vi "Process data first.vi"() -> ()   [LabVIEW 2021]
uses:
  <vilib>/Platform/TimedLoop/XDataNode/timing_clust.ctl
  <vilib>/Platform/TimedLoop/XDataNode/nitl_modes.ctl
  <vilib>/Platform/TimedLoop/XDataNode/wakeup.ctl
  <vilib>/picture/3D Picture Control/Object/Create Object (drawable).vi
  <vilib>/picture/3D Picture Control/Object/Add Object (no reference).vi
  <vilib>/picture/3D Picture Control/Object/Add Object (reference).vi
  <vilib>/platform/TimedLoop/XDataNode/XDataNode.xnode
  <vilib>/Platform/TimedLoop/XDataNode/XDNodeRunTimeDep.lvlib
  <vilib>/picture/3D Picture Control/NI_3D Picture Control.lvlib
panel:
  in  "Relative?":bool
  out "output variable 4":dbl
  out "Angle":dbl
  out "output variable 3":dbl
  out "output variable 2":dbl
  out "output variable":dbl
  out "3D Picture":refnum<vi>(3d-picture)
  out "ZRoll":dbl
  out "YRoll":dbl
  out "XRoll":dbl
  in  "stop":bool
  in  "DAQ Port":refnum<visa-resource-name>
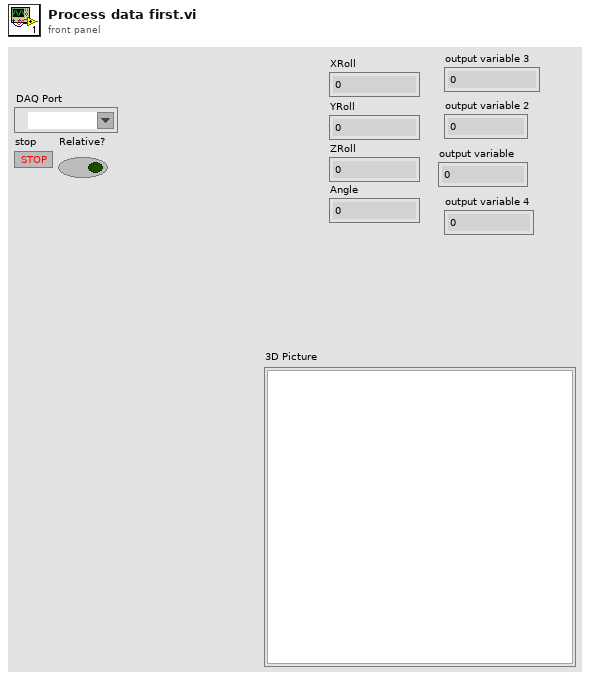
[diagram p1: front panel]
types:
  T1 = cluster{"Red":sgl, "Green":sgl, "Blue":sgl, "Alpha":sgl}
  T2 = typedef "XDNodeRunTimeDep.lvlib/timing_clust.ctl" = cluster{"Expected End [f-1]":u64, "Actual End [f-1]":u64, "Finished Late? [f-1]":bool, "Expected End [i-1]":u64, "Actual End [i-1]":u64, "Finished Late? [i-1]":bool, "Expected Start [i]":u64, "Actual Start [i]":u64, "Expected Start [f]":u64, "Actual Start [f]":u64, "Source Name":string, "Structure Name":string, "Period":i64, "Deadline":i64, "Offset":i64, "Start":i64, "Priority":i32, "Timeout":i32, "Mode":T3, "Wakeup Reason":T4, "Error":errorcluster, "Source Type":string, "Secondary Source Type":string, "Global End Time":u64, "Global Start Time":u64, "Frame Duration":u64, "Iteration Duration":u64, "Assigned CPU":i32, "I/O Scan Engine Mode":u32}
  T3 = typedef "XDNodeRunTimeDep.lvlib/nitl_modes.ctl" = enum32{"No Change", "Process missed periods, maintain original phase", "Discard missed periods, maintain original phase", "Process missed periods, ignore original phase", "Discard missed periods, ignore original phase"}
  T4 = typedef "XDNodeRunTimeDep.lvlib/wakeup.ctl" = enum32{"Normal", "Aborted", "Asynchronous wakeup", "Timing source error", "Timed loop error", "Timeout"}
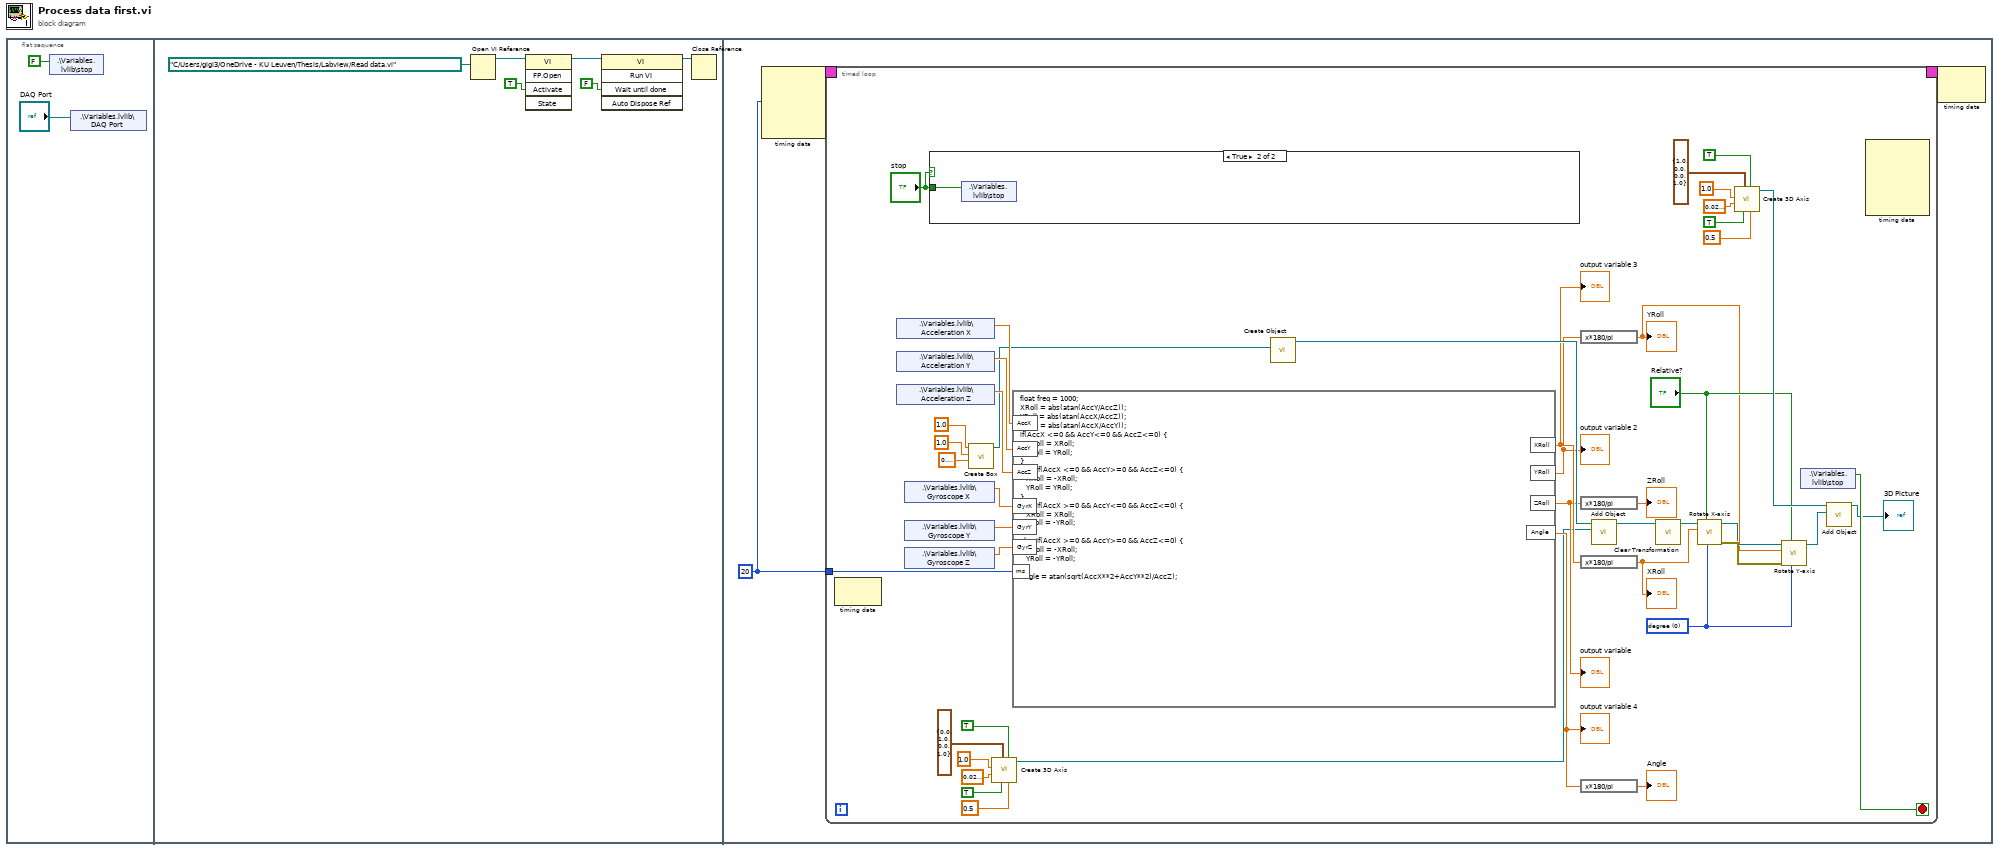
[diagram p0: block diagram]
diagram:
  n1 = flat-sequence {
    frame #0 {
      n2 = shared-variable ".\\Variables.lvlib\\stop"(FALSE ("stop")) -> ()  [unwired: 1 in, 1 out]
      n3 = shared-variable ".\\Variables.lvlib\\DAQ Port"("DAQ Port") -> ()  [unwired: 1 in, 1 out]
    }
    frame #1 {
      n4 = Open VI Reference(vi path=path "C:/Users/gigi3/OneDrive - KU Leuven/Thesis/Labview/Read data.vi") -> (vi reference=w8:refnum<vi>)  [unwired: 5 in, 1 out]
      n5 = invoke class="VI" method="FP.Open"(reference=w8, "Activate"=TRUE ("Activate?")) -> (reference out=w7:refnum<vi>)  [unwired: 3 in, 4 out]
      n6 = invoke class="VI" method="Run VI"(reference=w7, "Wait until done"=FALSE ("Wait Until Done")) -> (reference out=w4:refnum<vi>)  [unwired: 3 in, 4 out]
      n7 = Close Reference(reference=w4) -> ()  [unwired: 1 in, 1 out]
    }
    frame #2 {
      w9 = i64 20 ("Period")
      n8 = node-c288(w9) -> (w11:T2)  [unwired: 3 in]
      n9 = timed-loop {
        timing: w11 -> [_]
        timing-out: [_] -> w10
        tunnel: w9 -> [w47]
        stop <- w55 stop-if-true
        w12 = u16 0 items=["degree", "radians"] ("angle unit")
        n10 = node-c288() -> ()  [unwired: 1 in, 1 out]
        n11 = shared-variable ".\\Variables.lvlib\\Acceleration X"() -> (w53:dbl)  [unwired: 1 in, 1 out]
        n12 = shared-variable ".\\Variables.lvlib\\Acceleration Y"() -> (w52:dbl)  [unwired: 1 in, 1 out]
        n13 = shared-variable ".\\Variables.lvlib\\Acceleration Z"() -> (w51:dbl)  [unwired: 1 in, 1 out]
        n14 = shared-variable ".\\Variables.lvlib\\Gyroscope X"() -> (w50:dbl)  [unwired: 1 in, 1 out]
        n15 = shared-variable ".\\Variables.lvlib\\Gyroscope Y"() -> (w49:dbl)  [unwired: 1 in, 1 out]
        n16 = shared-variable ".\\Variables.lvlib\\Gyroscope Z"() -> (w48:dbl)  [unwired: 1 in, 1 out]
        n17 = case shown="True" "stop" {
          tunnel: "stop" -> [_ w58]
          frame False {
          }
          frame True {
            n18 = shared-variable ".\\Variables.lvlib\\stop"(w58) -> ()  [unwired: 1 in, 1 out]
          }
        }
        n19 = call <vilib>:"Create Box.vi"("Length Z"=sgl 0.1, "Length Y"=sgl 1.0, "Length X"=sgl 1.0) -> ("New Box Refnum"=w46:refnum<vi>)  [unwired: 7 in, 1 out]
        n20 = call <vilib>:"Create 3D Axis.vi"("Character Size"=sgl 0.5, "Half plane?"=TRUE, "Axis label?"=TRUE, "Color"=T1 {"Red"=0.0, "Green"=1.0, "Blue"=0.0, "Alpha"=1.0}, "Radius"=sgl 0.03, "Length"=sgl 1.0) -> ("New Object Refnum"=w29:refnum<vi>)  [unwired: 4 in, 1 out]
        n21 = formula code="float freq = 1000;\nXRoll = abs(atan(AccY/AccZ));\nYRoll = abs(atan(AccX/AccZ));\nZRoll = abs(atan(AccX/AccY));\nif(AccX <=0 && AccY<=0 && AccZ<=0) {\n   XRoll = XRoll;\n   YRoll = YRoll;\n}\nelse if(AccX <=0 && AccY>=0 && AccZ<=0) {\n   XRoll = -XRoll;\n   YRoll = YRoll;\n}\nelse if(AccX >=0 && AccY<=0 && AccZ<=0) {\n   XRoll = XRoll;\n   YRoll = -YRoll;\n}\nelse if(AccX >=0 && AccY>=0 && AccZ<=0) {\n   XRoll = -XRoll;\n   YRoll = -YRoll;\n}\nAngle = atan(sqrt(AccX**2+AccY**2)/AccZ);"("AccX"=w53, "AccY"=w52, "AccZ"=w51, "GyrX"=w50, "GyrY"=w49, "GyrZ"=w48, "ms"=w47) -> ("XRoll"=w33:dbl, "YRoll"=w32:dbl, "ZRoll"=w30:dbl, "Angle"=w31:dbl)
        "output variable" <- w30
        "output variable 2" <- w32
        "output variable 3" <- w33
        "output variable 4" <- w31
        n22 = call-poly <vilib>:"Create Object.vi"("Geometry"=w46) -> ("Scene:New Object"=w45:refnum<vi>)  [unwired: 9 in, 1 out]
        n23 = expression code="x*180/pi"(w32) -> (w15:dbl)
        "YRoll" <- w15
        n24 = expression code="x*180/pi"(w30) -> (→"ZRoll":dbl)
        n25 = expression code="x*180/pi"(w33) -> (w16:dbl)
        "XRoll" <- w16
        n26 = expression code="x*180/pi"(w31) -> (→"Angle":dbl)
        n27 = call-poly <vilib>:"Add Object.vi"("New Object In"=w29, "Scene Object In"=w45) -> ("Scene Object Out"=w14:refnum<vi>)  [unwired: 8 in, 1 out]
        n28 = call <vilib>:"Clear Transformation.vi"("Object Refnum In"=w14) -> ("Object Refnum Out"=w13:refnum<vi>)  [unwired: 9 in, 1 out]
        n29 = call <vilib>:"Rotate X-axis.vi"("angle unit"=w12, "Relative?"="Relative?", "angle"=w16, "Scene Object In"=w13) -> ("error out"=w21:errorcluster, "Scene Object Out"=w20:refnum<vi>)  [unwired: 6 in]
        n30 = call <vilib>:"Create 3D Axis.vi"("Character Size"=sgl 0.5, "Half plane?"=TRUE, "Axis label?"=TRUE, "Color"=T1 {"Red"=1.0, "Green"=0.0, "Blue"=0.0, "Alpha"=1.0}, "Radius"=sgl 0.03, "Length"=sgl 1.0) -> ("New Object Refnum"=w18:refnum<vi>)  [unwired: 4 in, 1 out]
        n31 = call <vilib>:"Rotate Y-axis.vi"("angle unit"=w12, "Relative?"="Relative?", "error in (no error)"=w21, "angle"=w15, "Scene Object In"=w20) -> ("Scene Object Out"=w19:refnum<vi>)  [unwired: 5 in, 1 out]
        n32 = shared-variable ".\\Variables.lvlib\\stop"() -> (w55:bool)  [unwired: 1 in, 1 out]
        n33 = call-poly <vilib>:"Add Object.vi"("New Object In"=w19, "Scene Object In"=w18) -> ("Scene Object Out"=→"3D Picture":refnum<vi>)  [unwired: 7 in, 2 out]
        n34 = node-c288() -> ()  [unwired: 5 in, 1 out]
      }
      n35 = node-c288(w10) -> ()  [unwired: 1 out]
    }
  }
